vi "ClassClearMutationHistory.vi"() -> ()   [LabVIEW 2020]
uses:
  <vilib>/Utility/EditLVLibs/Edit LVLibs.lvlib
panel:
  out "Path":path
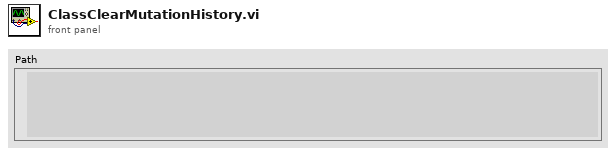
[diagram p1: front panel]
types:
  T1 = typedef "Edit LVLibs.lvlib/Mutation History.ctl" = T2[]
  T2 = typedef "Edit LVLibs.lvlib/Mutation Record.ctl" = cluster{"Library Version":T3, "Old Name Index":u8, "Class Default Data":variant, "Cluster Order Map":u32[], "Parent Name":string, "Parent Path":path, "LabVIEW Version":u32, "User Comments":string, "Mutation Flags":u8, "Parent Old Name Index":u8, "Parent Levels Added":u16, "Parent Levels Removed":u16}
  T3 = typedef "Edit LVLibs.lvlib/LibVersion.ctl" = cluster{"Major":u16, "Minor":u16, "Fix":u16, "Build":u16}
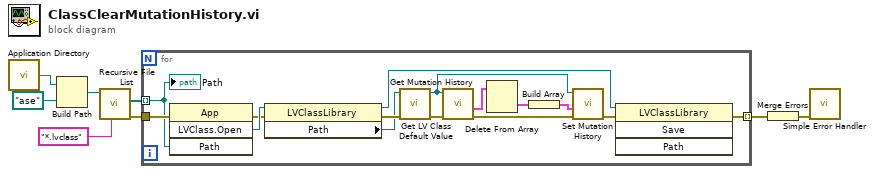
[diagram p0: block diagram]
diagram:
  n1 = call <vilib>:"Application Directory.vi"() -> ("Application Directory"=w8:path)
  n2 = Build Path(base path=w8, name or relative path=path "ase" ("base path")) -> (appended path=w2:path)
  n3 = call <vilib>:"Recursive File List.vi"("pattern"="*.lvclass", "Folder Path"=w2) -> ("error out"=w6:errorcluster, "All Files in Dir"=w5:path[])  [unwired: 5 in, 3 out]
  n4 = for {
    tunnel: w6 -> [w19]
    tunnel: w5 -> [w14] mode=indexing
    tunnel: [w11] -> w4 mode=indexing
    n5 = invoke class="App" method="LVClass.Open"(error in=w19, "Path"=w14) -> (error out=w17:errorcluster, "LVClass.Open"=w18:refnum<vi>)  [unwired: 2 in, 2 out]
    n6 = property class="LVClassLibrary"(reference=w18, error in=w17) -> (reference out=w12:refnum<vi>, error out=w16:errorcluster, "Path"=w15:path)
    n7 = call <vilib>:"Get LV Class Default Value.vi"("error in (no error)"=w16, "class path"=w15) -> ("error out"=w23:errorcluster, "object"=w20:refnum<class>)  [unwired: 8 in]
    n8 = call <vilib>:"Get Mutation History.vi"("error in"=w23, "Input object"=w20) -> ("error out"=w21:errorcluster, "Mutation History"=w22:T1)  [unwired: 6 in]
    n9 = Delete From Array(array=w22) -> (deleted portion=w10:T2)  [unwired: 2 in, 1 out]
    n10 = Build Array(w10) -> (w9:T2[])
    n11 = call <vilib>:"Set Mutation History.vi"("error in"=w21, "Mutation History"=w9, "Input object"=w20) -> ("error out"=w13:errorcluster)  [unwired: 8 in]
    n12 = invoke class="LVClassLibrary" method="Save"(reference=w12, error in=w13) -> (error out=w11:errorcluster)  [unwired: 2 in, 3 out]
    "Path" <- w14
  }
  n13 = Merge Errors(w4) -> (w3:errorcluster)
  n14 = call <vilib>:"Simple Error Handler.vi"("error in (no error)"=w3) -> ()  [unwired: 4 in, 5 out]
